vi "Do.vi"(8 "error in (no error)":errorcluster, 10 "Actor in":refnum<class "Actor.lvclass">, 11 "Increment2 Msg":refnum<class "Start Increment Msg.lvclass">) -> (0 "error out":errorcluster, 2 "Actor out":refnum<class "Actor.lvclass">)   [LabVIEW 2020, in "Messaging Tests.lvlib" / "Start Increment Msg.lvclass"]
uses:
  Start Increment Msg.lvclass
  Start Increment Msg.lvclass/Start Increment Msg.ctl
  Self Incrementer/Self Incrementer.lvclass
  vi.lib/ActorFramework/Actor/Actor.lvclass
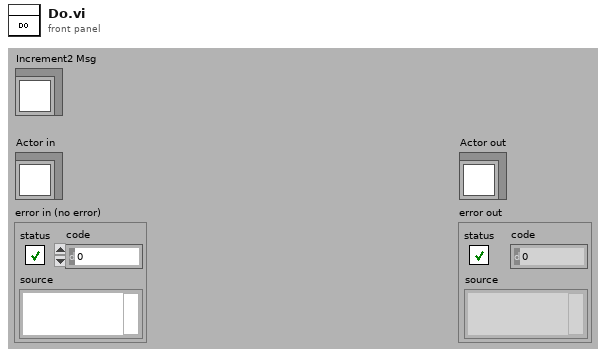
[diagram p1: front panel]
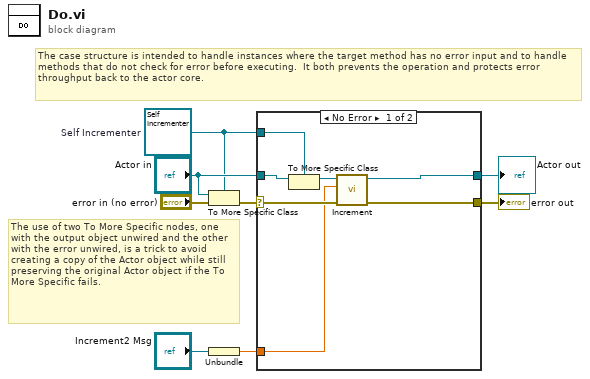
[diagram p0: block diagram]
diagram:
  w2 = refnum<class "Self Incrementer.lvclass"> refnum  # Self Incrementer
  # "The use of two To More Specific nodes, one with the output object unwired and the other with the error unwired, is a trick to avoid creating a copy of the Actor object while still preserving the original Actor object if the To More Specific fails."
  # "The case structure is intended to handle instances where the target method has no error input and to handle methods that do not check for error before executing.  It both prevents the operation and protects error throughput back to the actor core."
  n1 = To More Specific Class(target class=w2, reference="Actor in", error in="error in (no error)") -> (error out=w7:errorcluster)  [unwired: 1 out]
  n2 = Unbundle("Increment2 Msg") -> (w1:dbl)
  n3 = case shown="No Error" w7 {
    selector: w7 -> [w14 w17]
    tunnel: [w15 w17] -> w6
    tunnel: [w13 w16] -> w4
    tunnel: "Actor in" -> [w12 w16]
    tunnel: w2 -> [w11 _]
    tunnel: w1 -> [w9 _]
    frame No Error {
      n4 = To More Specific Class(target class=w11, reference=w12) -> (specific class reference=w10:refnum<class "Self Incrementer.lvclass">)  [unwired: 1 in, 1 out]
      n5 = call "Increment.vi"("error in (no error)"=w14, "Numeric"=w9, "TestActor in"=w10) -> ("error out"=w15:errorcluster, "TestActor out"=w13:refnum<class "Self Incrementer.lvclass">)  [unwired: 7 in]
    }
    frame Error {
      # "If type check fails, pass the original object out again."
    }
  }
  "error out" <- w6
  "Actor out" <- w4
